vi "Init UI.vi"(8 "error in (no error)":errorcluster, 11 "Deck in":refnum<class "Deck.lvclass">) -> (0 "error out":errorcluster, 3 "Deck out":refnum<class "Deck.lvclass">)   [LabVIEW 2019, in "Deck.lvclass"]
uses:
  Deck.lvclass
  Packed Libraries/Messaging.lvlibp
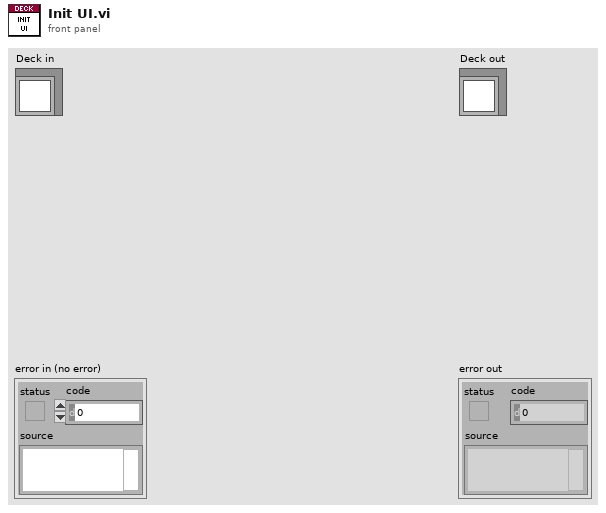
[diagram p1: front panel]
types:
  T1 = typedef "Audio Processing.lvlibp/Value Properties.ctl" = cluster{"Lower":dbl, "Upper":dbl, "Default":dbl, "Increment":dbl}
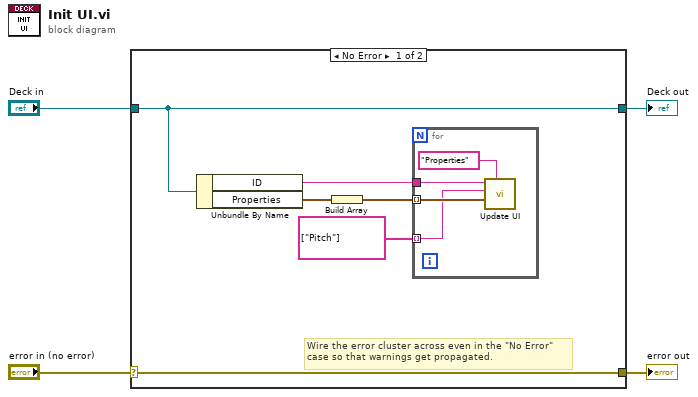
[diagram p0: block diagram]
diagram:
  n1 = case shown="No Error" "error in (no error)" {
    selector: "error in (no error)" -> [w10 w16]
    tunnel: [w10 w16] -> w3
    tunnel: [w9 w15] -> w1
    tunnel: "Deck in" -> [w9 w15]
    frame No Error {
      # "Wire the error cluster across even in the \"No Error\"\ncase so that warnings get propagated."
      n2 = Unbundle By Name(w9) -> ("ID"=w8:string, "Properties"=w7:T1)
      n3 = Build Array(w7) -> (w6:T1[])
      n4 = for {
        tunnel: w8 -> [w14]
        tunnel: w6 -> [w13] mode=indexing
        tunnel: string[] ["Pitch"] -> [w12] mode=indexing
        n5 = call "Update UI.vi"("Message (Value Change)"="Properties", "Data"=w13, "Target"=w12, "ID"=w14) -> ()  [unwired: 7 in, 1 out]
      }
    }
    frame Error {
    }
  }
  "error out" <- w3
  "Deck out" <- w1
